vi "AlliGator Get Python Plugin Functions List.vi"(8 "Error In":errorcluster, 9 "Include Example Plugins":bool, 11 "Python Plugins Folder Path":path) -> (0 "Error Out":errorcluster, 3 "Array of Python Functions":T1[](array[typedef]))   [LabVIEW 2021, in "AlliGator Python Plugins.lvlib"]
doc: "Extracts list of python plugin functions from the Python Plugin folder."
uses:
  AlliGator Python Plugins.lvlib
  AlliGator Python Function Information.ctl
  AlliGator Python Function Parameter Definition.ctl
  AlliGator Python Function Output Definition.ctl
  AlliGator Python Plugin Target Type.ctl
panel:
  # "see the AlliGator License on the block diagram (Ctrl+E or Window:Show Block Diagram)"
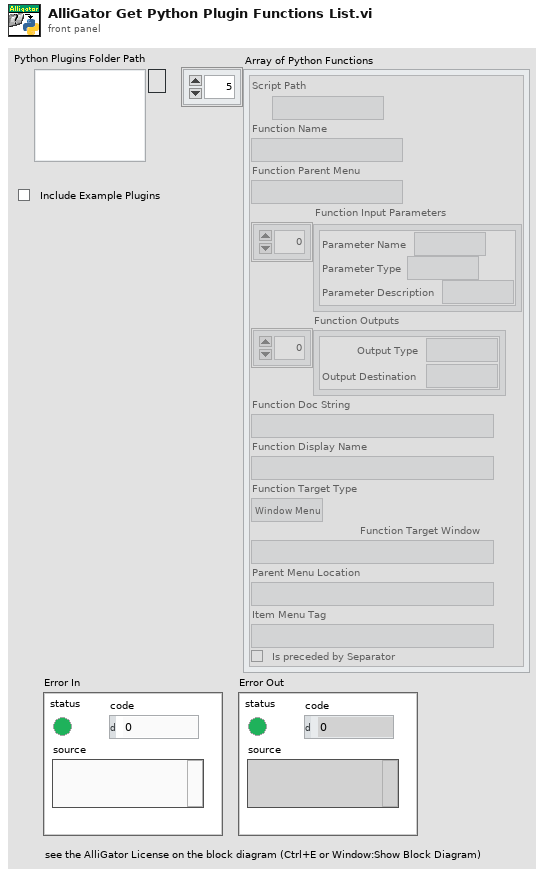
[diagram p1: front panel]
types:
  T1 = typedef "AlliGator Python Plugins.lvlib/AlliGator Python Function Information.ctl" = cluster{"Script Path":path, "Function Name":string, "Function Parent Menu":string, "Function Input Parameters":T2[], "Function Outputs":T3[], "Function Doc String":string, "Function Display Name":string, "Function Target Type":T4, "Function Target Window":string, "Parent Menu Location":string, "Item Menu Tag":string, "Is preceded by Separator":bool}
  T2 = typedef "AlliGator Python Plugins.lvlib/AlliGator Python Function Parameter Definition.ctl" = cluster{"Parameter Name":string, "Parameter Type":string, "Parameter Description":string}
  T3 = typedef "AlliGator Python Plugins.lvlib/AlliGator Python Function Output Definition.ctl" = cluster{"Output Type":string, "Output Destination":string}
  T4 = typedef "AlliGator Python Plugins.lvlib/AlliGator Python Plugin Target Type.ctl" = enum16{"Undefined", "Window Menu", "Object Menu"}
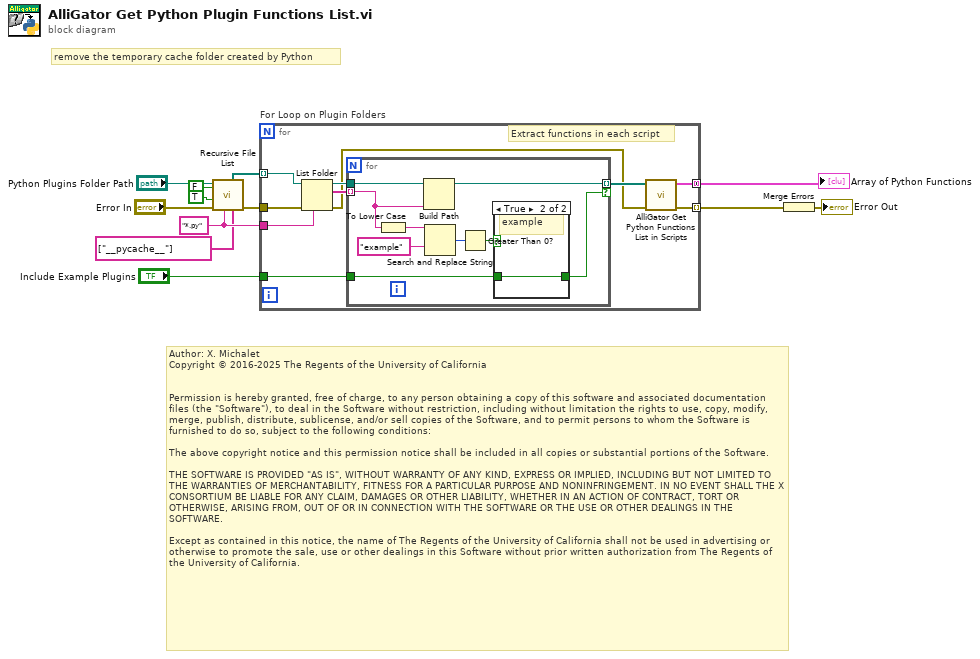
[diagram p0: block diagram]
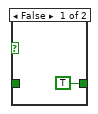
[diagram p2: hidden frame]
diagram:
  w7 = "*.py" ("pattern")
  # "Author: X. Michalet\nCopyright © 2016-2025 The Regents of the University of California\n \n\nPermission is hereby granted, free of charge, to any person obtaining a copy of this software and associated documentation files (the \"Software\"), to deal in the Software without restriction, including without limitation the rights to use, copy, modify, merge, publish, distribute, sublicense, and/or sell copies of the Software, and to permit persons to whom the Software is furnished to do so, subject to the following conditions:\n\nThe above copyright notice and this permission notice shall be included in all copies or substantial portions of the Software.\n\nTHE SOFTWARE IS PROVIDED \"AS IS\", WITHOUT WARRANTY OF ANY KIND, EXPRESS OR IMPLIED, INCLUDING BUT NOT LIMITED TO THE WARRANTIES OF MERCHANTABILITY, FITNESS FOR A PARTICULAR PURPOSE AND NONINFRINGEMENT. IN NO EVENT SHALL THE X CONSORTIUM BE LIABLE FOR ANY CLAIM, DAMAGES OR OTHER LIABILITY, WHETHER IN AN ACTION OF CONTRACT, TORT OR OTHERWISE, ARISING FROM, OUT OF OR IN CONNECTION WITH THE SOFTWARE OR THE USE OR OTHER DEALINGS IN THE SOFTWARE.\n\nExcept as contained in this notice, the name of The Regents of the University of California shall not be used in advertising or otherwise to promote the sale, use or other dealings in this Software without prior written authorization from The Regents of the University of California."
  # "remove the temporary cache folder created by Python"
  n1 = call <vilib>:"Recursive File List.vi"("Folders to Exclude"=string[] ["__pycache__"], "pattern"=w7, "error in (no error)"="Error In", "Continue Recursing on Error? (F)"=TRUE, "Treat LLBs as Folders?"=FALSE, "Folder Path"="Python Plugins Folder Path") -> ("error out"=w8:errorcluster, "All Folders"=w4:path[])  [unwired: 1 in, 3 out]
  n2 = for "For Loop on Plugin Folders" {
    tunnel: w4 -> [w22] mode=indexing
    tunnel: w7 -> [w20]
    tunnel: [w17] -> w3 mode=concatenating
    tunnel: w8 -> [w21]
    tunnel: [w18] -> w6 mode=indexing
    tunnel: "Include Example Plugins" -> [w16]
    # "Extract functions in each script"
    n3 = List Folder(path=w22, pattern=w20, error in=w21) -> (path out=w15:path, filenames=w14:string[], error out=w13:errorcluster)  [unwired: 1 in, 1 out]
    n4 = for {
      tunnel: w15 -> [w31]
      tunnel: w14 -> [w29] mode=indexing
      tunnel: [w30] -> w19 mode=indexing if=w23
      tunnel: w16 -> [w24]
      n5 = To Lower Case(string=w29) -> (all lower case string=w27:string)
      n6 = Build Path(base path=w31, name or relative path=w29) -> (appended path=w30:path)
      n7 = Search and Replace String(input string=w27, search string="example") -> (number of replacements=w26:i32)  [unwired: 6 in, 3 out]
      n8 = Greater Than 0?(x=w26) -> (x > 0?=w25:bool)
      n9 = case shown="True" w25 {
        tunnel: w24 -> [_ w33]
        tunnel: [TRUE ("Include Example Plugins") w33] -> w23
        frame False {
        }
        frame True {
          # "example"
        }
      }
    }
    n10 = call "AlliGator Get Python Functions List in Scripts.vi"("error in (no error)"=w13, "All Files in Dir"=w19) -> ("error out"=w18:errorcluster, "Array of Python Functions"=w17:T1[])  [unwired: 7 in, 1 out]
  }
  "Array of Python Functions" <- w3
  n11 = Merge Errors(w6) -> (→"Error Out":errorcluster)
